vi "GetRoutineDefinitionFromController.vi"(0 "System no.":i32=1 min=1 max=4 step=1, 1 "Fast Routine type":enum16{"FDG", "FDR"}(ring), 5 "error in":errorcluster) -> (15 "Routine Definitons":string, 19 "error out":errorcluster)   [LabVIEW 2020]
doc: "This VI uses FRR? to query all fast routine definitions from controller and diplays them as text string.\nRoutine definitions can either be FDG (Gradient Search Scan) or FDR (Area Scan Routine)."
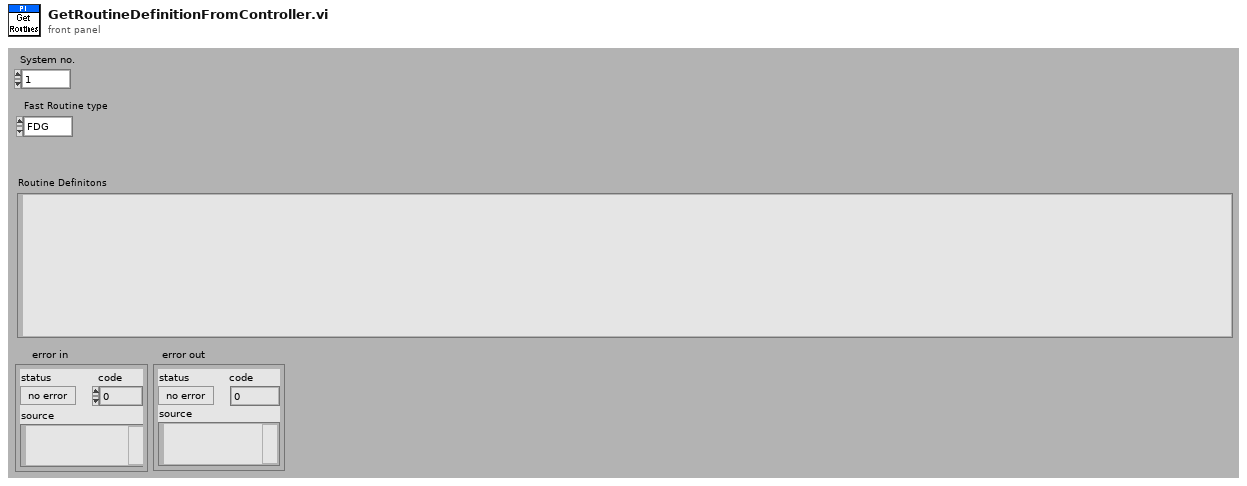
[diagram p1: front panel]
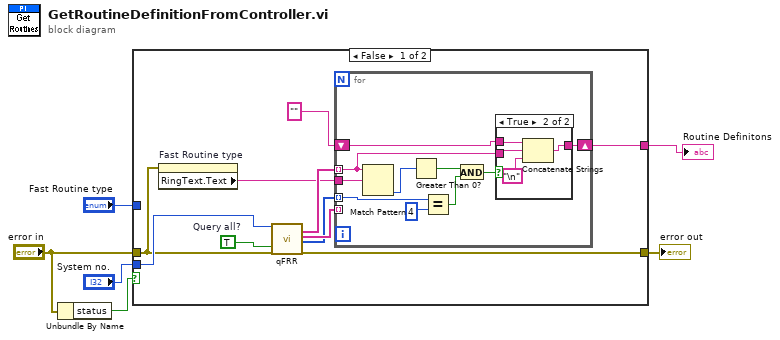
[diagram p0: block diagram]
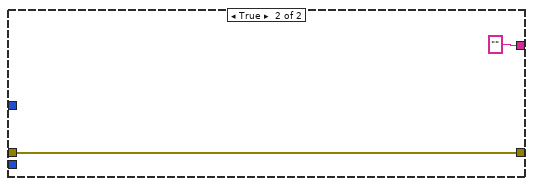
[diagram p3: hidden frame]
diagram:
  n1 = Unbundle By Name("error in") -> ("status"=w4:bool)
  n2 = case shown="False" w4 {
    tunnel: "System no." -> [w16 _]
    tunnel: "error in" -> [w13 w33]
    tunnel: [w14 w33] -> w3
    tunnel: "Fast Routine type" -> [_ _]
    tunnel: [w8 ""] -> w1
    frame False {
      w15 = TRUE  # Query all?
      n3 = property on="Fast Routine type" class="Enum (strict)"(error in=w13) -> ("RingText.Text"=w9:string)  [unwired: 1 in, 2 out]
      n4 = call "qFRR.vi"("System no."=w16, "Query all?"=w15, "error in"=w13) -> ("Value (string)"=w12:string[], "Queried routinename out"=w11:string[], "ResultID out"=w10:i32[], "error out"=w14:errorcluster)  [unwired: 3 in, 10 out]
      n5 = for {
        tunnel: w12 -> [w18] mode=indexing
        tunnel: w11 -> [_] mode=indexing
        tunnel: w10 -> [w26] mode=indexing
        tunnel: w9 -> [w24]
        shift-right: [w17] -> w8
        shift-left: "" -> [w19]
        n6 = Match Pattern(string=w18, regular expression=w24) -> (offset past match=w23:i32)  [unwired: 4 out]
        n7 = Greater Than 0?(x=w23) -> (x > 0?=w22:bool)
        n8 = Equal?(x=w26, y=4) -> (x = y?=w21:bool)
        n9 = And(x=w22, y=w21) -> (x .and. y?=w20:bool)
        n10 = case shown="True" w20 {
          tunnel: w19 -> [w27 w31]
          tunnel: w18 -> [_ w29]
          tunnel: [w27 w30] -> w17
          frame False {
          }
          frame True {
            n11 = Concatenate Strings(w31, w29, "\n") -> (w30:string)
          }
        }
      }
    }
    frame True {
    }
  }
  "error out" <- w3
  "Routine Definitons" <- w1
